vi "Request PropertyObject.vi"(7 "Type":T1, 8 "error in (no error)":errorcluster, 9 "Lookup String":string, 10 "Scope":refnum<class "PropertyObject.lvclass">, 11 "Engine in":refnum<class "Engine.lvclass">) -> (0 "error out":errorcluster, 2 "PropertyObject":refnum<class "PropertyObject.lvclass">)   [LabVIEW 2020, in "TSnax.lvlib" / "Engine.lvclass"]
uses:
  Engine.lvclass
  Engine.lvclass/Engine.ctl
  PropertyObject/PropertyObject.lvclass
  VariableContainer Response.ctl
  VariableContainer Type.ctl
  VariableContainer Request.ctl
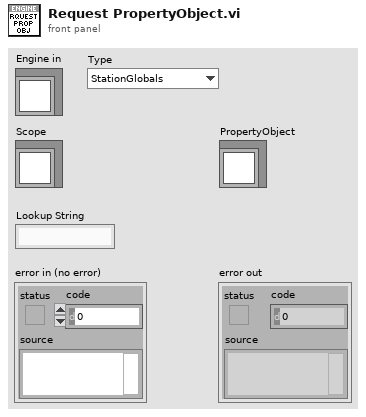
[diagram p1: front panel]
types:
  T1 = typedef "TSnax.lvlib/Engine.lvclass/VariableContainer Type.ctl" = enum16{"StationGlobals", "TemporaryGlobals", "NewPropertyObject", "SubProperty"}
  T2 = typedef "TSnax.lvlib/Engine.lvclass/VariableContainer Request.ctl" = cluster{"Type":T1, "Scope":refnum<class "PropertyObject.lvclass">, "Lookup String":string, "Notifier":refnum<notifier>}
  T3 = typedef "TSnax.lvlib/Engine.lvclass/VariableContainer Response.ctl" = cluster{"PropertyObject":refnum<class "PropertyObject.lvclass">, "Error":errorcluster}
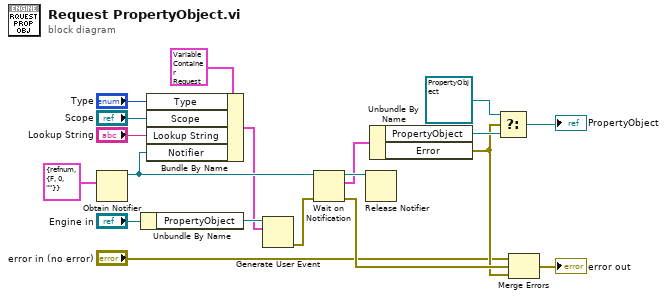
[diagram p0: block diagram]
diagram:
  n1 = Obtain Notifier(notification data type=T3 {"PropertyObject"=refnum, "Error"={"status"=FALSE, "code"=0, "source"=""}} ("VariableContainer Response")) -> (notifier out=w7:refnum<notifier>)  [unwired: 3 in, 2 out]
  n2 = Unbundle By Name("Engine in") -> ("PropertyObject"=w16:refnum<user-event>)
  n3 = Bundle By Name(cluster=T2 {"Type"=enum."StationGlobals", "Scope"=refnum, "Lookup String"="", "Notifier"=refnum} ("VariableContainer Request"), "Type"="Type", "Scope"="Scope", "Lookup String"="Lookup String", "Notifier"=w7) -> (w1:T2)
  n4 = Generate User Event(user event=w16, event data cluster=w1) -> (error out=w19:errorcluster)  [unwired: 2 in, 1 out]
  n5 = Wait on Notification(notifier=w7, error in (no error)=w19) -> (notifier out=w14:refnum<notifier>, notification=w13:T3, error out=w12:errorcluster)  [unwired: 2 in, 1 out]
  n6 = Release Notifier(notifier=w14) -> ()  [unwired: 2 in, 3 out]
  n7 = Unbundle By Name(w13) -> ("PropertyObject"=w15:refnum<class "PropertyObject.lvclass">, "Error"=w11:errorcluster)
  n8 = Select(t=refnum<class "PropertyObject.lvclass"> refnum, s=w11, f=w15) -> (s? t:f=→"PropertyObject":refnum<class "PropertyObject.lvclass">)
  n9 = Merge Errors("error in (no error)", w12, w11) -> (→"error out":errorcluster)
